vi "Agilent B2900 Series Output List Sweep Volts.vi"() -> ()   [LabVIEW 2023]
doc: "This example shows how to use the instrument's output voltage sweep list mode. The actual voltage levels and actual current levels are returned as well as whether over current protection (OCP) has been tripped."
uses:
  Agilent B2900 Series.lvlib
  Public/Data/Low Level/Fetch Measurement (Multiple Points).vi
  Public/Configure/Measurement/Configure Measurement (Current).vi
panel:
  in  "Compliance Current (0.0001 A)":dbl=0.0001
  in  "Voltage List":dbl[](array[numeric])
  in  "Current NPLC (0.1)":dbl=0.1
  in  "Trigger Source (0: Auto-Internal)":i32(ring) items=["Auto-Internal", "Bus", "Timer", "INT1", "INT2", "LAN", "EXT1", "EXT2", "EXT3", "EXT4", "EXT5", "EXT6", "EXT7", "EXT8", "EXT9", "EXT10", "EXT11", "EXT12", "EXT13", "EXT14"]
  in  "Enable Output Protection (T: Enable)":bool=TRUE
  out "OCP Tripped?":bool
  out "Actual Current Levels (A)":dbl[](array[numeric])
  out "Actual Voltage Levels (V)":dbl[](array[numeric])
  in  "Channel (0: Channel 1)":i32(ring) items=["Channel 1", "Channel 2"]
  in  "VISA resource name":refnum<visa-resource-name>
  # "(c) 2011-2021 National Instruments.  ALL RIGHTS RESERVED."
  # "Compliance Protection"
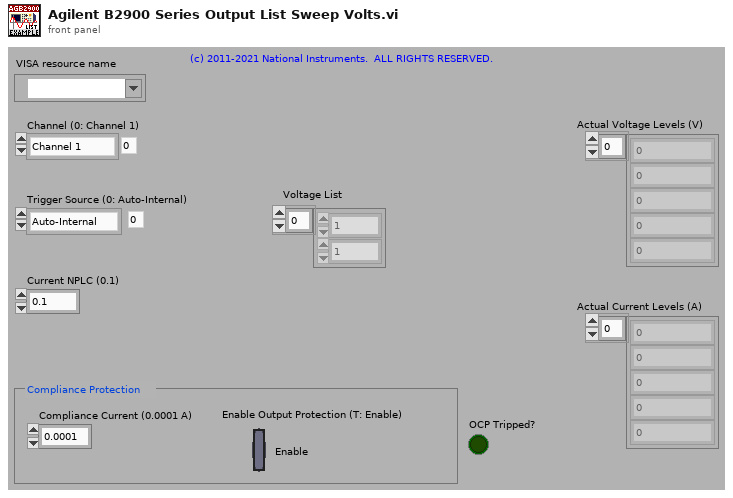
[diagram p1: front panel]
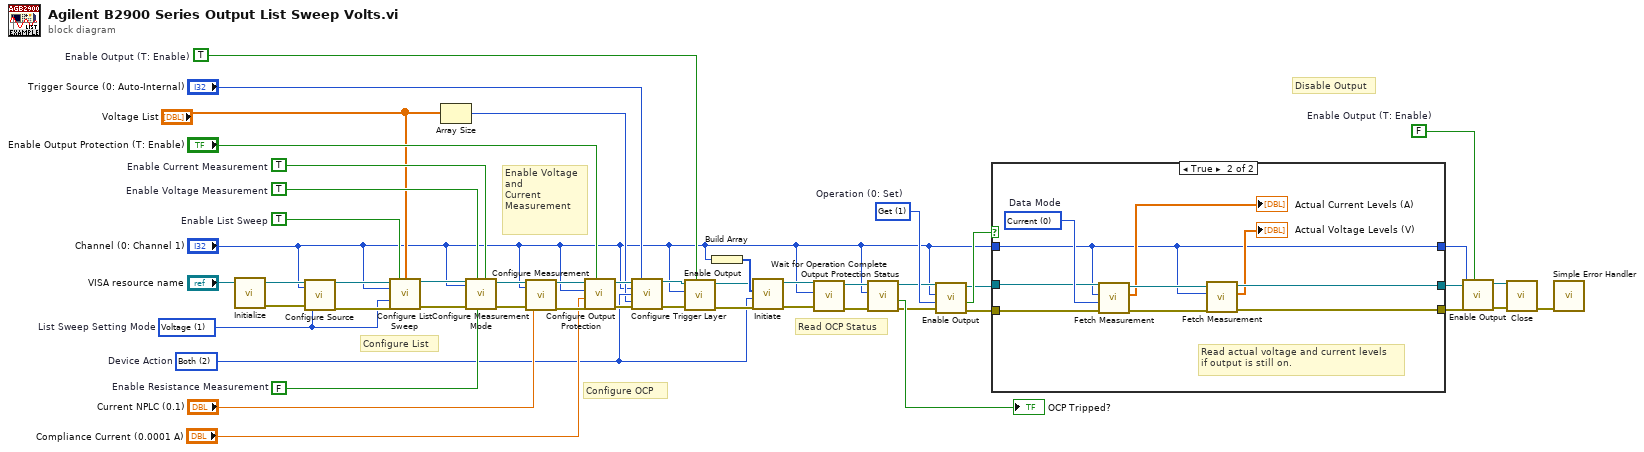
[diagram p0: block diagram]
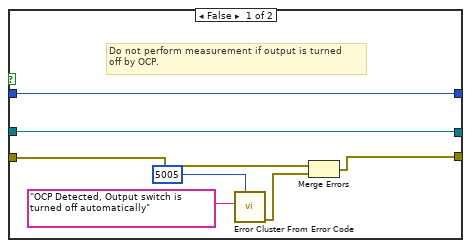
[diagram p2: hidden frame]
diagram:
  w16 = 1 items=["Set", "Get"]  # Operation (0: Set)
  w23 = TRUE  # Enable Current Measurement
  w24 = TRUE  # Enable Voltage Measurement
  w38 = FALSE  # Enable Output (T: Enable)
  w4 = 2 items=["Acquire", "Transient", "Both"]  # Device Action
  w45 = FALSE  # Enable Resistance Measurement
  w20 = 1 items=["Current", "Voltage"]  # List Sweep Setting Mode
  w19 = TRUE  # Enable List Sweep
  w43 = TRUE  # Enable Output (T: Enable)
  # "Configure List"
  # "Disable Output"
  # "Read OCP Status"
  # "Enable Voltage and \nCurrent Measurement"
  # "Configure OCP"
  n1 = call "Initialize.vi"("VISA resource name"="VISA resource name") -> ("error out"=w21:errorcluster, "VISA resource name out"=w22:refnum<visa-resource-name>)  [unwired: 9 in]
  n2 = call "Configure Source.vi"("VISA resource name"=w22, "Channel (0: Channel 1)"="Channel (0: Channel 1)", "error in (no error)"=w21, "Source Mode (1: Voltage)"=w20) -> ("VISA resource name out"=w33:refnum<visa-resource-name>, "error out"=w32:errorcluster)  [unwired: 14 in]
  n3 = call "Configure List Sweep.vi"("VISA resource name"=w33, "Enable List Sweep (F: Disable)"=w19, "Sweep List Data"="Voltage List", "Channel (0: Channel 1)"="Channel (0: Channel 1)", "List Sweep Setting Mode (1: Voltage)"=w20, "error in (no error)"=w32) -> ("VISA resource name out"=w26:refnum<visa-resource-name>, "error out"=w25:errorcluster)  [unwired: 8 in]
  n4 = Array Size(array="Voltage List") -> (size(s)=w3:i32)
  n5 = call "Configure Measurement Mode.vi"("Enable Current Measurement (T: Enable)"=w23, "Enable Resistance Measurement (F: Disable)"=w45, "Enable Voltage Measurement (T: Enable)"=w24, "error in (no error)"=w25, "Channel (0: Channel 1)"="Channel (0: Channel 1)", "VISA resource name"=w26) -> ("error out"=w30:errorcluster, "VISA resource name out"=w31:refnum<visa-resource-name>)  [unwired: 4 in]
  n6 = call-poly "Configure Measurement.vi"("VISA resource name"=w31, "Channel (0: Channel 1)"="Channel (0: Channel 1)", "error in (no error)"=w30, "Current NPLC (0.1)"="Current NPLC (0.1)") -> ("VISA resource name out"=w28:refnum<visa-resource-name>, "error out"=w27:errorcluster)  [unwired: 14 in]
  n7 = call "Configure Output Protection.vi"("Enable Output Protection (T: Enable)"="Enable Output Protection (T: Enable)", "error in (no error)"=w27, "Compliance Current (0.0001 A)"="Compliance Current (0.0001 A)", "Channel (0: Channel 1)"="Channel (0: Channel 1)", "VISA resource name"=w28) -> ("error out"=w7:errorcluster, "VISA resource name out"=w8:refnum<visa-resource-name>)  [unwired: 5 in]
  n8 = call "Configure Trigger Layer.vi"("VISA resource name"=w8, "Trigger Source (0: Auto-Internal)"="Trigger Source (0: Auto-Internal)", "Channel (0: Channel 1)"="Channel (0: Channel 1)", "Device Action (2: Both)"=w4, "Trigger Count (1)"=w3, "error in (no error)"=w7) -> ("VISA resource name out"=w5:refnum<visa-resource-name>, "error out"=w6:errorcluster)  [unwired: 8 in]
  n9 = call "Enable Output.vi"("Enable Output (F: Disable)"=w43, "error in (no error)"=w6, "Channel (0: Channel 1)"="Channel (0: Channel 1)", "VISA resource name"=w5) -> ("error out"=w39:errorcluster, "VISA resource name out"=w40:refnum<visa-resource-name>)  [unwired: 5 in, 1 out]
  n10 = Build Array("Channel (0: Channel 1)") -> (w46:i32[])
  n11 = call "Initiate.vi"("error in (no error)"=w39, "Device Action (2: Both)"=w4, "Channel List ({Channel1})"=w46, "VISA resource name"=w40) -> ("error out"=w36:errorcluster, "VISA resource name out"=w37:refnum<visa-resource-name>)  [unwired: 6 in]
  n12 = call "Wait for Operation Complete.vi"("error in (no error)"=w36, "Channel (0: Channel 1)"="Channel (0: Channel 1)", "VISA resource name"=w37) -> ("error out"=w34:errorcluster, "VISA resource name out"=w35:refnum<visa-resource-name>)  [unwired: 7 in]
  n13 = call "Output Protection Status.vi"("error in (no error)"=w34, "Channel (0: Channel 1)"="Channel (0: Channel 1)", "VISA resource name"=w35) -> ("error out"=w11:errorcluster, "OCP Tripped?"=→"OCP Tripped?":bool, "VISA resource name out"=w13:refnum<visa-resource-name>)  [unwired: 5 in, 1 out]
  n14 = call "Enable Output.vi"("error in (no error)"=w11, "Operation (0: Set)"=w16, "Channel (0: Channel 1)"="Channel (0: Channel 1)", "VISA resource name"=w13) -> ("error out"=w12:errorcluster, "Output Enabled?"=w15:bool, "VISA resource name out"=w14:refnum<visa-resource-name>)  [unwired: 5 in]
  n15 = case shown="True" w15 {
    tunnel: [w57 w67] -> w42
    tunnel: [w51 w66] -> w41
    tunnel: w14 -> [w57 w60]
    tunnel: w12 -> [w52 w59]
    tunnel: "Channel (0: Channel 1)" -> [w56 w58]
    tunnel: [w56 w58] -> w17
    frame False {
      # "Do not perform measurement if output is turned\noff by OCP."
      n16 = call <vilib>:"Error Cluster From Error Code.vi"("error message (\"\")"="OCP Detected, Output switch is turned off automatically" ("error message (\"\")"), "error code (0)"=5005) -> ("error out"=w53:errorcluster)  [unwired: 7 in]
      n17 = Merge Errors(w52, w53) -> (w51:errorcluster)
    }
    frame True {
      w61 = 0 items=["Current", "Resistance", "Source Output Setting", "Status", "Time", "Voltage"]  # Data Mode
      # "Read actual voltage and current levels \nif output is still on."
      n18 = call-poly "Fetch Measurement.vi"("error in (no error)"=w59, "Data Mode (5: Voltage)"=w61, "Channel (0: Channel 1)"=w58, "VISA resource name"=w60) -> ("error out"=w62:errorcluster, "Measurements"=→"Actual Current Levels (A)":dbl[], "VISA resource name out"=w64:refnum<visa-resource-name>)  [unwired: 5 in]
      n19 = call-poly "Fetch Measurement.vi"("error in (no error)"=w62, "Channel (0: Channel 1)"=w58, "VISA resource name"=w64) -> ("error out"=w66:errorcluster, "Measurements"=→"Actual Voltage Levels (V)":dbl[], "VISA resource name out"=w67:refnum<visa-resource-name>)  [unwired: 6 in]
    }
  }
  n20 = call "Enable Output.vi"("Enable Output (F: Disable)"=w38, "error in (no error)"=w41, "Channel (0: Channel 1)"=w17, "VISA resource name"=w42) -> ("error out"=w47:errorcluster, "VISA resource name out"=w48:refnum<visa-resource-name>)  [unwired: 5 in, 1 out]
  n21 = call "Close.vi"("error in (no error)"=w47, "VISA resource name"=w48) -> ("error out"=w49:errorcluster)  [unwired: 9 in]
  n22 = call <vilib>:"Simple Error Handler.vi"("error in (no error)"=w49) -> ()  [unwired: 4 in, 5 out]
